vi "Naming Check.vi"(8 "error in (no error)":errorcluster, 11 "Name (\"\" to Use UUID)":string) -> (0 "error out":errorcluster, 3 "Name (Dup)":string)   [LabVIEW 2017, in "Communicable State Machine.lvlib"]
doc: "### Naming Check.vi\n\n-- <b>Controls</b> --\n- <b>Name(\"\" to use uuid)</b>:\nReturns any argument(s) that may be used in the current state string. These arguments come after the \">>\" characters\n\n-- <b>Indicators</b> --\n- <b>Name(dup)</b>:\nReturns any argument(s) that may be used in the current state string. These arguments come after the \">>\" characters"
uses:
  Communicable State Machine.lvlib
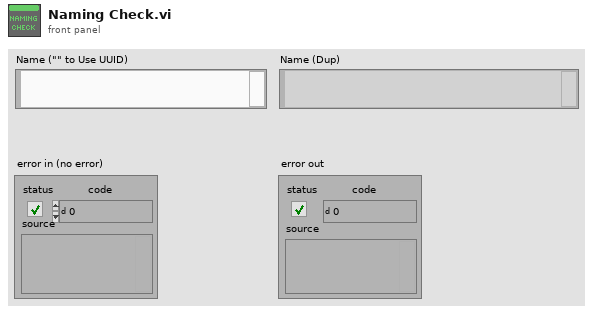
[diagram p1: front panel]
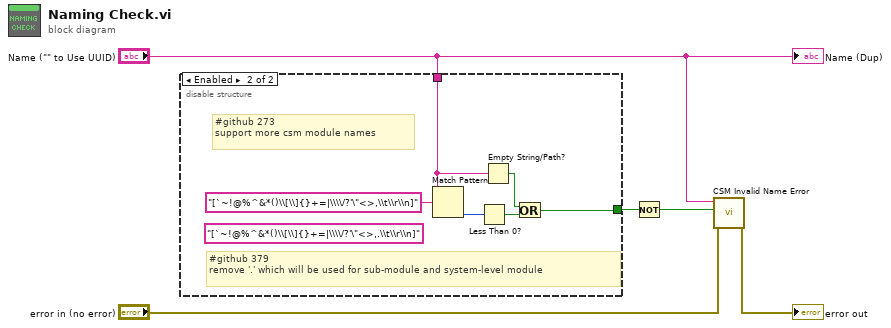
[diagram p0: block diagram]
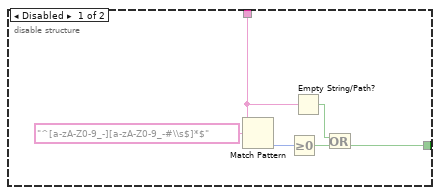
[diagram p2: hidden frame]
diagram:
  n1 = disable-structure shown="Enabled" {
    disable-tunnel: "Name (\"\" to Use UUID)" -> [w8 w12]
    disable-tunnel: [w7 w13] -> w2
    frame Disabled {
      n2 = Match Pattern(string=w8, regular expression="^[a-zA-Z0-9_-][a-zA-Z0-9_-#\\s$]*$") -> (offset past match=w10:i32)  [unwired: 1 in, 3 out]
      n3 = Greater Or Equal To 0?(x=w10) -> (x >= 0?=w9:bool)
      n4 = Empty String/Path?(string/path=w8) -> (empty?=w6:bool)
      n5 = Or(x=w6, y=w9) -> (x .or. y?=w7:bool)
    }
    frame Enabled {
      (unwired) "[`~!@%^&*()\\[\\]{}+=|\\\\/?'\"<>,.\\t\\r\\n]" ("regular expression")
      # "#github 379 \nremove '.' which will be used for sub-module and system-level module"
      # "#github 273 \nsupport more csm module names"
      n6 = Match Pattern(string=w12, regular expression="[`~!@%^&*()\\[\\]{}+=|\\\\/?'\"<>,\\t\\r\\n]") -> (offset past match=w16:i32)  [unwired: 1 in, 3 out]
      n7 = Less Than 0?(x=w16) -> (x < 0?=w15:bool)
      n8 = Empty String/Path?(string/path=w12) -> (empty?=w14:bool)
      n9 = Or(x=w14, y=w15) -> (x .or. y?=w13:bool)
    }
  }
  n10 = Not(x=w2) -> (.not. x?=w1:bool)
  n11 = call "CSM Invalid Name Error.vi"("error in (no error)"="error in (no error)", "Occured"=w1, "Name (\"\" to Use UUID)"="Name (\"\" to Use UUID)") -> ("error out"=→"error out":errorcluster)  [unwired: 8 in]
  "Name (Dup)" <- "Name (\"\" to Use UUID)"
